vi "Set X Maximum.vi"(9 "Waveform Reference Cluster":T1, 11 "Display Size":T2(ring)) -> ()   [LabVIEW 2014]
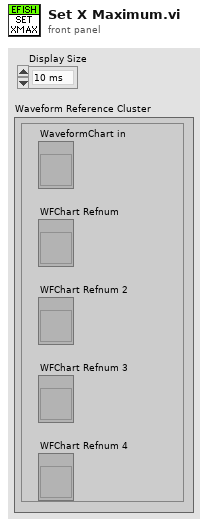
[diagram p1: front panel]
types:
  T1 = cluster{"WFChart Refnum":refnum<vi>, "WFChart Refnum 2":refnum<vi>, "WFChart Refnum 3":refnum<vi>, "WFChart Refnum 4":refnum<vi>, "WaveformChart in":refnum<vi>}
  T2 = enum16{"10 ms", "100 ms", "1 Second", "10 sec", "30 sec"}
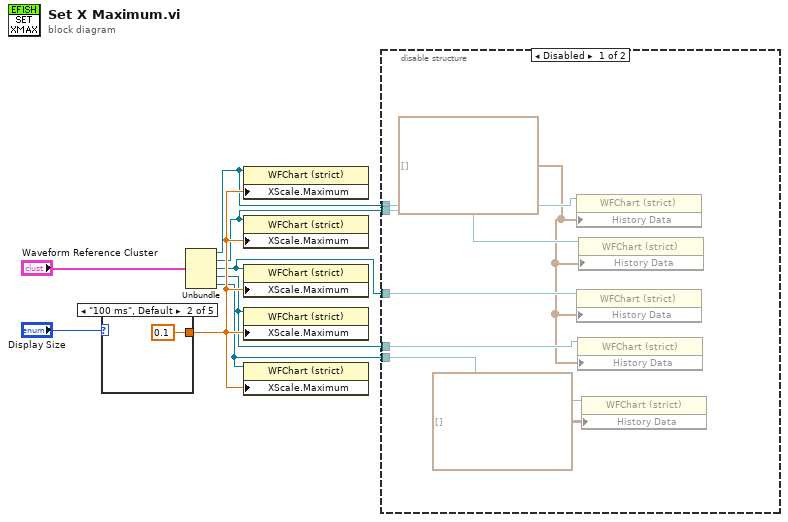
[diagram p0: block diagram]
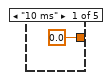
[diagram p3: hidden frame]
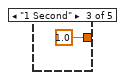
[diagram p4: hidden frame]
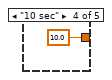
[diagram p5: hidden frame]
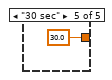
[diagram p6: hidden frame]
diagram:
  n1 = case shown="\"100 ms\", Default" "Display Size" {
    tunnel: [0.0 0.1 1.0 10.0 30.0] -> w8
    frame "10 ms" {
    }
    frame "100 ms", Default {
    }
    frame "1 Second" {
    }
    frame "10 sec" {
    }
    frame "30 sec" {
    }
  }
  n2 = Unbundle("Waveform Reference Cluster") -> ("WFChart Refnum"=w5:refnum<vi>, "WFChart Refnum 2"=w4:refnum<vi>, "WFChart Refnum 3"=w3:refnum<vi>, "WFChart Refnum 4"=w2:refnum<vi>, "WaveformChart in"=w1:refnum<vi>)
  n3 = property on="Property Node" class="WFChart (strict)"(reference=w5, "XScale.Maximum"=w8) -> ()  [unwired: 1 in, 2 out]
  n4 = property on="Property Node" class="WFChart (strict)"(reference=w4, "XScale.Maximum"=w8) -> ()  [unwired: 1 in, 2 out]
  n5 = property on="Property Node" class="WFChart (strict)"(reference=w3, "XScale.Maximum"=w8) -> ()  [unwired: 1 in, 2 out]
  n6 = property on="Property Node" class="WFChart (strict)"(reference=w2, "XScale.Maximum"=w8) -> ()  [unwired: 1 in, 2 out]
  n7 = property on="Property Node" class="WFChart (strict)"(reference=w1, "XScale.Maximum"=w8) -> ()  [unwired: 1 in, 2 out]
  n8 = disable-structure shown="Disabled" {
    disable-tunnel: w5 -> [w20 _]
    disable-tunnel: w4 -> [w19 _]
    disable-tunnel: w3 -> [w18 _]
    disable-tunnel: w2 -> [w17 _]
    disable-tunnel: w1 -> [w16 _]
    frame Disabled {
      w15 = waveform(dbl)[] [] ("History Data")
      n9 = property on="Property Node" class="WFChart (strict)"(reference=w20, "History Data"=w15) -> ()  [unwired: 1 in, 2 out]
      n10 = property on="Property Node" class="WFChart (strict)"(reference=w18, "History Data"=w15) -> ()  [unwired: 1 in, 2 out]
      n11 = property on="Property Node" class="WFChart (strict)"(reference=w17, "History Data"=w15) -> ()  [unwired: 1 in, 2 out]
      n12 = property on="Property Node" class="WFChart (strict)"(reference=w19, "History Data"=w15) -> ()  [unwired: 1 in, 2 out]
      n13 = property on="Property Node" class="WFChart (strict)"(reference=w16, "History Data"=waveform(dbl)[][] []) -> ()  [unwired: 1 in, 2 out]
    }
    frame Enabled {
    }
  }
